vi "仁科测控RS-KTC-N01温湿度解析.vi"(11 "运行状态输入":u16[](array[numeric])) -> (3 "温湿度解析":cluster{"湿度":dbl, "温度":dbl})   [LabVIEW 2016, in "环境动力监测库.lvlib" / "空调库.lvlib"]
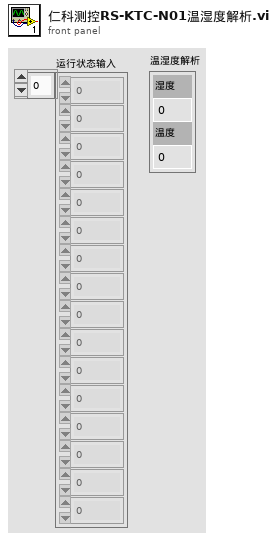
[diagram p1: front panel]
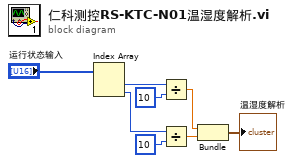
[diagram p0: block diagram]
diagram:
  n1 = Index Array(array="运行状态输入") -> (element #1=w6:u16, element #2=w3:u16)  [unwired: 2 in]
  n2 = Divide(x=w6, y=u16 10) -> (x/y=w2:dbl)
  n3 = Divide(x=w3, y=u16 10) -> (x/y=w1:dbl)
  n4 = Bundle(w2, w1) -> (→"温湿度解析":cluster{dbl, dbl})  [unwired: 1 in]
